vi "Configure Jitter Trend.vi"(0 "VISA resource name":refnum<visa-resource-name>, 1 "Enable Jitter Trend (T: Enable)":bool=TRUE, 2 "Auto Vertical Mode  (T: Enable)":bool=TRUE, 5 "Offset (0 s)":dbl, 7 "Range (4E-9 s)":dbl=4e-09, 9 "Smooth Points (5)":dbl=5.0, 11 "error in (no error)":errorcluster, 12 "Enable Trend Smoothing (T: Enable)":bool=TRUE) -> (4 "VISA resource name out":refnum<visa-resource-name>, 15 "error out":errorcluster)   [LabVIEW 2020, in "Agilent 90000 Series.lvlib"]
doc: "Configures measurement trend analysis and its parameters."
uses:
  Agilent 90000 Series.lvlib
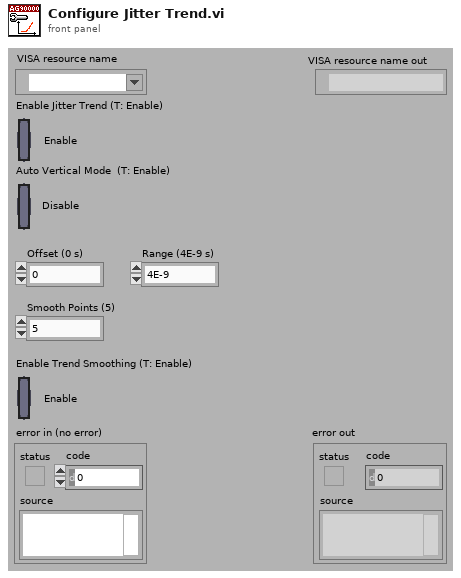
[diagram p1: front panel]
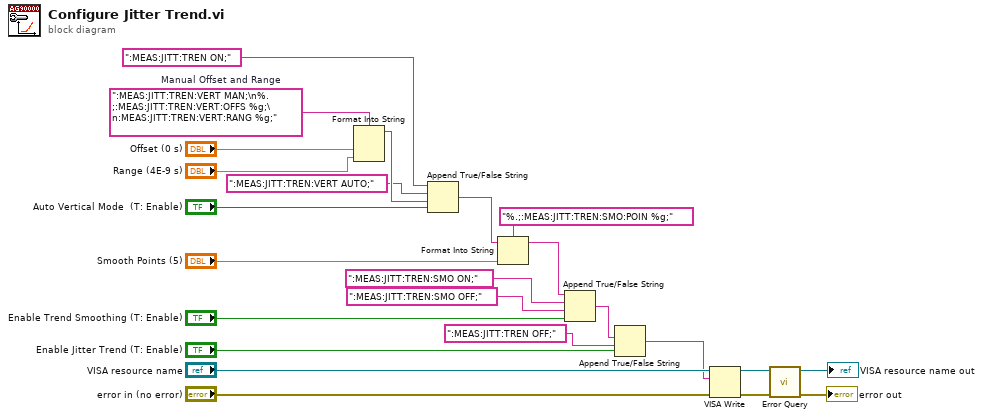
[diagram p0: block diagram]
diagram:
  w15 = ":MEAS:JITT:TREN:VERT MAN;\n%.;:MEAS:JITT:TREN:VERT:OFFS %g;\n:MEAS:JITT:TREN:VERT:RANG %g;"  # Manual Offset and Range
  n1 = Format Into String(format string=w15, "Offset (0 s)", "Range (4E-9 s)") -> (resulting string=w14:string)  [unwired: 2 in, 1 out]
  n2 = Append True/False String(1:"Auto Vertical Mode  (T: Enable)", 2:w14, 3:":MEAS:JITT:TREN:VERT AUTO;" ("true string"), 4:":MEAS:JITT:TREN ON;" ("initial string")) -> (0:w9:string)
  n3 = Format Into String(format string="%.;:MEAS:JITT:TREN:SMO:POIN %g;", initial string=w9, "Smooth Points (5)") -> (resulting string=w7:string)  [unwired: 1 in, 1 out]
  n4 = Append True/False String(1:"Enable Trend Smoothing (T: Enable)", 2:":MEAS:JITT:TREN:SMO OFF;" ("false string"), 3:":MEAS:JITT:TREN:SMO ON;" ("true string"), 4:w7) -> (0:w5:string)
  n5 = Append True/False String(1:"Enable Jitter Trend (T: Enable)", 2:":MEAS:JITT:TREN OFF;" ("initial string"), 3:w5) -> (0:w2:string)  [unwired: 1 out]
  n6 = VISA Write(VISA resource name="VISA resource name", write buffer=w2, error in (no error)="error in (no error)") -> (VISA resource name out=w23:refnum<visa-resource-name>, error out=w20:errorcluster)  [unwired: 1 out]
  n7 = call "Error Query.vi"("error in (no error)"=w20, "VISA resource name"=w23) -> ("error out"=→"error out":errorcluster, "VISA resource name out"=→"VISA resource name out":refnum<visa-resource-name>)  [unwired: 8 out]
